vi "GetText.vi"(8 "error in":errorcluster, 11 "tag bus configurable plugin editor node in":refnum<class "tag bus processing plugin editor node.lvclass">) -> (0 "error out":errorcluster, 1 "additional text":string, 2 "text":string, 3 "tag bus configurable plugin editor node out":refnum<class "tag bus processing plugin editor node.lvclass">, 4 "glyph":string)   [LabVIEW 2013, in "tag bus processing plugin editor node.lvclass"]
uses:
  tag bus processing plugin editor node.lvclass
  <vilib>/NI/Tag Bus Data Framework/Configuration Editor/Classes/Module editor node/Read display name.vi
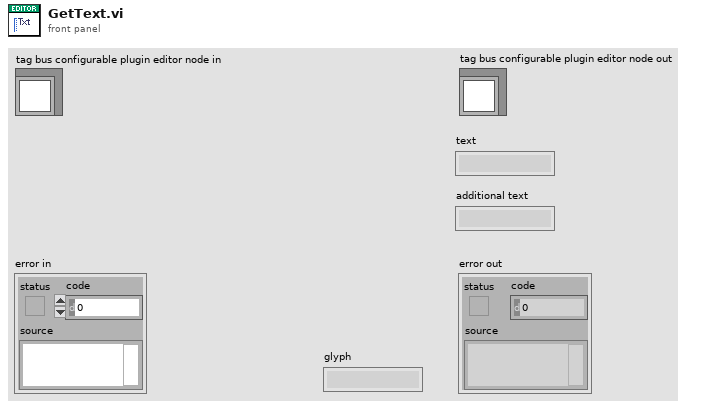
[diagram p1: front panel]
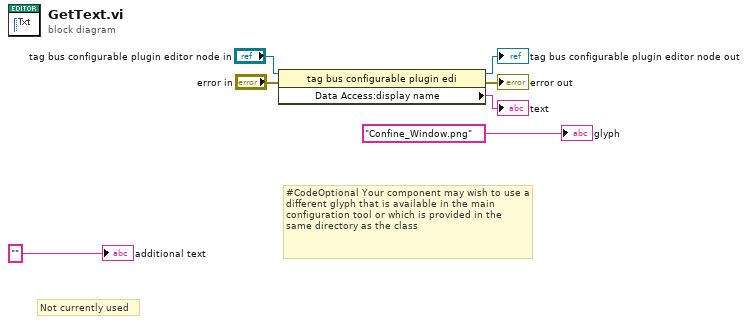
[diagram p0: block diagram]
diagram:
  # "Not currently used"
  # "#CodeOptional Your component may wish to use a different glyph that is available in the main configuration tool or which is provided in the same directory as the class"
  n1 = property class="tag bus configurable plugin edi"(reference="tag bus configurable plugin editor node in", error in="error in") -> (reference out=→"tag bus configurable plugin editor node out":refnum<class "tag bus processing plugin editor node.lvclass">, error out=→"error out":errorcluster, "Data Access:display name"=→"text":string)
  "additional text" <- "" ("additional text")
  "glyph" <- "Confine_Window.png" ("glyph")
